vi "Read Channel C of XY.vi"(6 "Y":dbl[](array[numeric]), 9 "X":dbl[](array[numeric]), 10 "C":i32[](array[numeric]), 11 "Channel Chosen":i32) -> (0 "Last entry from channel C?":bool, 2 "Y":dbl[](array[numeric]), 3 "X":dbl[](array[numeric]))   [LabVIEW 2023]
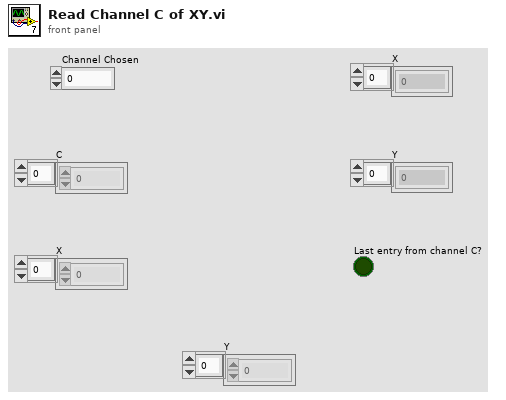
[diagram p1: front panel]
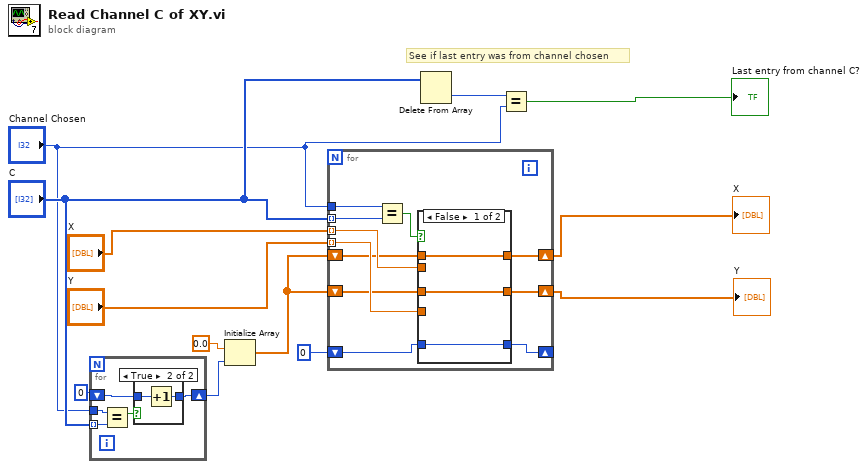
[diagram p0: block diagram]
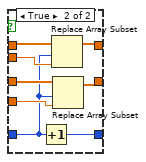
[diagram p3: hidden frame]
diagram:
  # "See if last entry was from channel chosen"
  n1 = for {
    tunnel: "C" -> [w17] mode=indexing
    tunnel: "Channel Chosen" -> [w18]
    shift-right: [w14] -> w6
    shift-left: 0 -> [w15]
    n2 = Equal?(x=w18, y=w17) -> (x = y?=w16:bool)
    n3 = case shown="True" w16 {
      tunnel: w15 -> [w19 w21]
      tunnel: [w19 w20] -> w14
      frame False {
      }
      frame True {
        n4 = Increment(x=w21) -> (x+1=w20:i32)
      }
    }
  }
  n5 = Initialize Array(0.0 ("element"), w6) -> (w4:dbl[])
  n6 = for {
    tunnel: "C" -> [w32] mode=indexing
    tunnel: "X" -> [w30] mode=indexing
    tunnel: "Y" -> [w29] mode=indexing
    tunnel: "Channel Chosen" -> [w26]
    shift-right: [w25] -> w2
    shift-left: w4 -> [w27]
    shift-right: [w24] -> w3
    shift-left: w4 -> [w28]
    shift-right: [w22] -> _
    shift-left: 0 -> [w23]
    n7 = Equal?(x=w26, y=w32) -> (x = y?=w31:bool)
    n8 = case shown="False" w31 {
      tunnel: w30 -> [_ w39]
      tunnel: w29 -> [_ w41]
      tunnel: [w35 w43] -> w24
      tunnel: [w34 w42] -> w25
      tunnel: w28 -> [w35 w40]
      tunnel: w27 -> [w34 w38]
      tunnel: w23 -> [w33 w36]
      tunnel: [w33 w37] -> w22
      frame False {
      }
      frame True {
        n9 = Increment(x=w36) -> (x+1=w37:i32)
        n10 = Replace Array Subset(array=w40, new element=w39, index=w36) -> (w43:dbl[])
        n11 = Replace Array Subset(array=w38, new element=w41, index=w36) -> (w42:dbl[])
      }
    }
  }
  "Y" <- w2
  "X" <- w3
  n12 = Delete From Array(array="C") -> (deleted portion=w11:i32)  [unwired: 2 in, 1 out]
  n13 = Equal?(x=w11, y="Channel Chosen") -> (x = y?=→"Last entry from channel C?":bool)
